vi "Replace Element.vi"(7 "element name":string, 8 "error in":errorcluster, 10 "value":variant, 11 "cluster in":variant) -> (0 "error out":errorcluster, 3 "cluster out":variant)   [LabVIEW 2020, in "PV Access.lvlib" / "PV Data.lvlib"]
uses:
  PV Data.lvlib
  <userlib>/_OpenG.lib/lvdata/lvdata.llb/openg_variant.lvlib
  Error Codes.ctl
  <userlib>/_OpenG.lib/error/error.llb/openg_error.lvlib
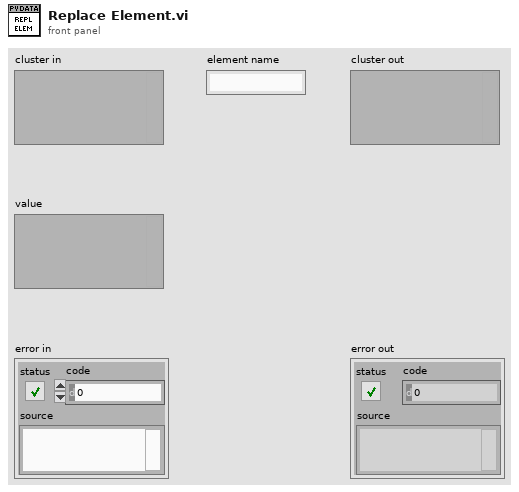
[diagram p1: front panel]
types:
  T1 = typedef "openg_variant.lvlib/Type Descriptor Enumeration__ogtk.ctl" = enum8{"<Null>", "I8", "I16", "I32", "I64", "U8", "U16", "U32", "U64", "SGL", "DBL", "EXT", "CSG", "CDB", "CXT", "0x0F", "0x10", "0x11", "0x12", "0x13", "0x14", "Enum U8", "Enum U16", "Enum U32", "Enum U64", "SGL PQ", "DBL PQ", "EXT PQ", "CSG PQ", "CDB PQ", "CXT PQ", "0x1F", "0x20", "Boolean", "0x22", "0x23", "0x24", "0x25", "0x26", "0x27", "0x28", "0x29", "0x2A", "0x2B", "0x2C", "0x2D", "0x2E", "0x2F", "String", "0x31", "Path", "Pict", "0x34", "0x35", "0x36", "DAQ", "0x38", "0x39", "0x3A", "0x3B", "0x3C", "0x3D", "0x3E", "0x3F", "Array", "0x41", "0x42", "0x43", "0x44", "0x45", "0x46", "0x47", "0x48", "0x49", "0x4A", "0x4B", "0x4C", "0x4D", "0x4E", "0x4F", "Cluster", "0x51", "0x52", "Variant", "Waveform", "0x55", "0x56", "0x57", "0x58", "0x59", "0x5A", "0x5B", "0x5C", "0x5D", "0x5E", "Fixed Point", "0x60", "0x61", "0x62", "0x63", "0x64", "0x65", "0x66", "0x67", "0x68", "0x69", "0x6A", "0x6B", "0x6C", "0x6D", "0x6E", "0x6F", "Refnum", "0x71", "0x72", "Set Collection", "Map Collection"}
  T2 = typedef "PV Access.lvlib/PV Data.lvlib/Error Codes.ctl" = i32
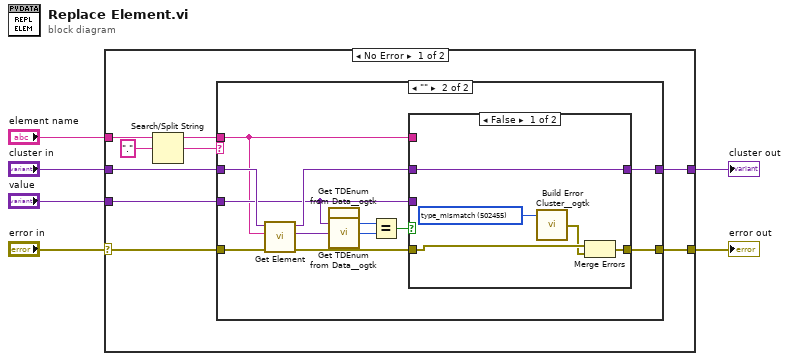
[diagram p0: block diagram]
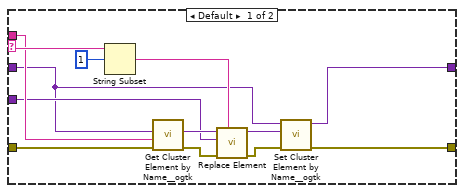
[diagram p2: hidden frame]
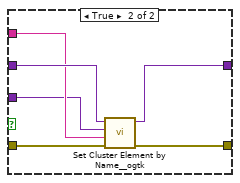
[diagram p3: hidden frame]
diagram:
  n1 = case shown="No Error" "error in" {
    selector: "error in" -> [w13 w53]
    tunnel: [w15 w53] -> w2
    tunnel: "element name" -> [w9 _]
    tunnel: "cluster in" -> [w12 w52]
    tunnel: "value" -> [w11 _]
    tunnel: [w14 w52] -> w3
    frame No Error {
      n2 = Search/Split String(string=w9, search string/char (-)=".") -> (substring before match=w8:string, match + rest of string=w7:string)  [unwired: 1 in, 1 out]
      n3 = case shown="\"\"" w7 {
        selector: w7 -> [w26 _]
        tunnel: [w20 w40] -> w15
        tunnel: [w16 w39] -> w14
        tunnel: w13 -> [w25 w35]
        tunnel: w12 -> [w17 w33]
        tunnel: w11 -> [w21 w30]
        tunnel: w8 -> [w23 w29]
        frame Default {
          n4 = String Subset(string=w26, offset (0)=1) -> (substring=w27:string)  [unwired: 1 in]
          n5 = call <userlib>:"Get Cluster Element by Name__ogtk.vi"("error in (no error)"=w25, "Element Name"=w23, "Cluster"=w17) -> ("error out"=w24:errorcluster, "VElement"=w22:variant)  [unwired: 6 in, 1 out]
          n6 = call "Replace Element.vi"("element name"=w27, "error in"=w24, "value"=w21, "cluster in"=w22) -> ("error out"=w19:errorcluster, "cluster out"=w18:variant)  [unwired: 6 in]
          n7 = call <userlib>:"Set Cluster Element by Name__ogtk.vi"("error in (no error)"=w19, "New Element Value"=w18, "Cluster"=w17) -> ("error out"=w20:errorcluster, "VCluster out"=w16:variant)  [unwired: 6 in, 1 out]
        }
        frame "" {
          n8 = call "Get Element.vi"("error in"=w35, "element name"=w29, "cluster in"=w33) -> ("error out"=w34:errorcluster, "element"=w31:variant, "cluster out"=w32:variant)  [unwired: 6 in]
          n9 = call <userlib>:"Get TDEnum from Data__ogtk.vi"("Data"=w30) -> ("Type Descriptor Enumeration"=w37:T1)  [unwired: 4 in]
          n10 = call <userlib>:"Get TDEnum from Data__ogtk.vi"("Data"=w31) -> ("Type Descriptor Enumeration"=w38:T1)  [unwired: 4 in]
          n11 = Equal?(x=w37, y=w38) -> (x = y?=w36:bool)
          n12 = case shown="False" w36 {
            tunnel: [w45 w51] -> w40
            tunnel: [w41 w50] -> w39
            tunnel: w34 -> [w44 w49]
            tunnel: w29 -> [_ w47]
            tunnel: w32 -> [w41 w48]
            tunnel: w30 -> [_ w46]
            frame False {
              w43 = T2 502455 items=["unspecified"=502450, "interrupted"=502451, "timeout"=502452, "field_missing"=502453, "cannot_convert_value"=502454, "type_mismatch"=502455] ("Ring")
              n13 = call <userlib>:"Build Error Cluster__ogtk.vi"("code"=w43) -> ("error out"=w42:errorcluster)  [unwired: 1 in]
              n14 = Merge Errors(w44, w42) -> (w45:errorcluster)
            }
            frame True {
              n15 = call <userlib>:"Set Cluster Element by Name__ogtk.vi"("error in (no error)"=w49, "Element Name (\"\": New Element Data Name)"=w47, "New Element Value"=w46, "Cluster"=w48) -> ("error out"=w51:errorcluster, "VCluster out"=w50:variant)  [unwired: 5 in, 1 out]
            }
          }
        }
      }
    }
    frame Error {
    }
  }
  "error out" <- w2
  "cluster out" <- w3
